vi "writeToXML.vi"(8 "error in (no error)":errorcluster, 10 "ClassLabel":string, 11 "AbsorbPOrigin in":refnum<class "AbsorbPOrigin.lvclass">) -> (0 "error out":errorcluster, 2 "XML out":string, 3 "AbsorbPOrigin out":refnum<class "AbsorbPOrigin.lvclass">)   [LabVIEW 2014, in "TCSDataDefinitions.lvlib" / "TCSCommand.lvlib" / "POriginCommands.lvlib" / "AbsorbPOrigin.lvclass"]
uses:
  AbsorbPOrigin.lvclass
  AbsorbPOrigin.lvclass/AbsorbPOrigin.ctl
  POriginCommands/POriginCommands.lvclass
  <userlib>/Common/XML/XMLGenerator/XMLGenerator.lvclass
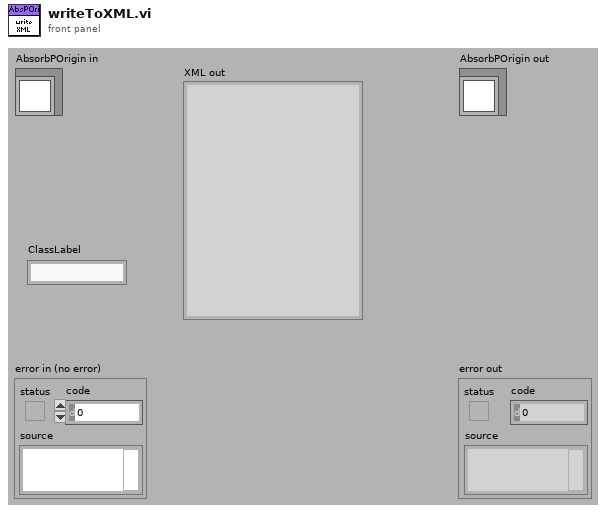
[diagram p1: front panel]
types:
  T1 = typedef "TCSDataDefinitions.lvlib/TCSCommand.lvlib/OffsetCommands.lvlib/Num2Types.ctl" = enum16{"User", "Handset", "Both"}
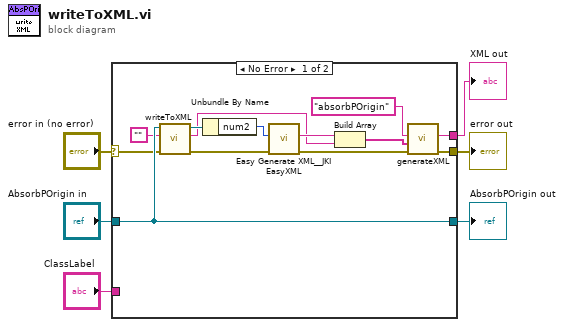
[diagram p0: block diagram]
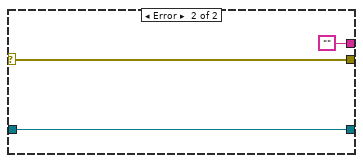
[diagram p2: hidden frame]
diagram:
  n1 = case shown="No Error" "error in (no error)" {
    selector: "error in (no error)" -> [w11 w22]
    tunnel: [w10 w22] -> w5
    tunnel: [w18 w21] -> w3
    tunnel: "AbsorbPOrigin in" -> [w18 w21]
    tunnel: [w7 ""] -> w2
    tunnel: "ClassLabel" -> [_ _]
    frame No Error {
      n2 = call-parent "writeToXML.vi"("error in (no error)"=w11, "ClassLabel"="", "POriginCommands in"=w18) -> ("error out"=w15:errorcluster, "XML out"=w13:string, "POriginCommands out"=w17:refnum<class "AbsorbPOrigin.lvclass">)  [unwired: 6 in]
      n3 = Unbundle By Name(w17) -> ("num2"=w19:T1)
      n4 = call <vilib>:"Easy Generate XML__JKI EasyXML.vi"("error in (no error)"=w15, "LabVIEW Data"=w19) -> ("error out"=w12:errorcluster, "XML String"=w14:string)  [unwired: 8 in]
      n5 = Build Array(w14, w13) -> (w9:string[])
      n6 = call <userlib>:"generateXML.vi"("error in"=w12, "childrenXML"=w9, "elementName"="absorbPOrigin" ("Class Label")) -> ("error out"=w10:errorcluster, "XML out"=w7:string)  [unwired: 6 in, 1 out]
    }
    frame Error {
    }
  }
  "error out" <- w5
  "AbsorbPOrigin out" <- w3
  "XML out" <- w2
